vi "Insert.vi"(8 "error in (no error)":errorcluster caption="错误输入（无错误）", 11 "Access User 输入":refnum<class "Access User.lvclass">) -> (0 "error out":errorcluster caption="错误输出", 2 "字符串":string, 3 "Access User 输出":refnum<class "Access User.lvclass">)   [LabVIEW 2017, in "Access User.lvclass"]
uses:
  Access User.lvclass
  Abstract User/Abstract User.lvclass
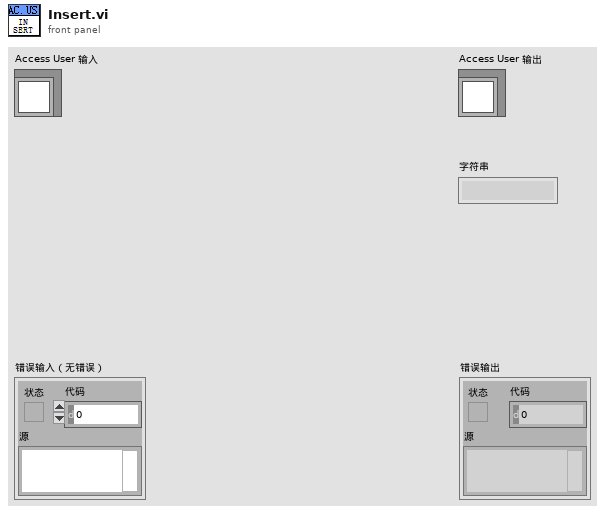
[diagram p1: front panel]
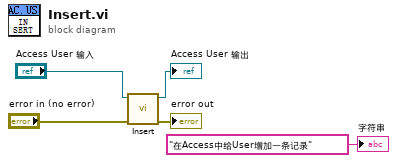
[diagram p0: block diagram]
diagram:
  n1 = call-parent "Insert.vi"("error in (no error)"="error in (no error)", "Abstract User 输入"="Access User 输入") -> ("error out"=→"error out":errorcluster, "Abstract User 输出"=→"Access User 输出":refnum<class "Access User.lvclass">)  [unwired: 7 in, 1 out]
  "字符串" <- "在Access中给User增加一条记录" ("字符串")
